vi "io_unit.vi"(0 "from_alu":T1, 1 "from_regs":T1, 2 "from_input":T1, 3 "to":T1, 4 "from":T1) -> (5 "to_alu":T2, 6 "to_regs":T2, 7 "to_output":T2)   [LabVIEW 2013]
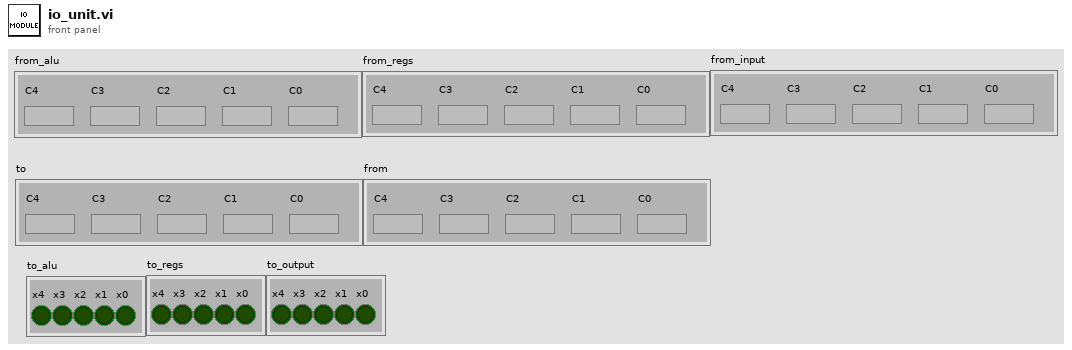
[diagram p1: front panel]
types:
  T1 = cluster{"C4":bool, "C3":bool, "C2":bool, "C1":bool, "C0":bool}
  T2 = cluster{"x4":bool, "x3":bool, "x2":bool, "x1":bool, "x0":bool}
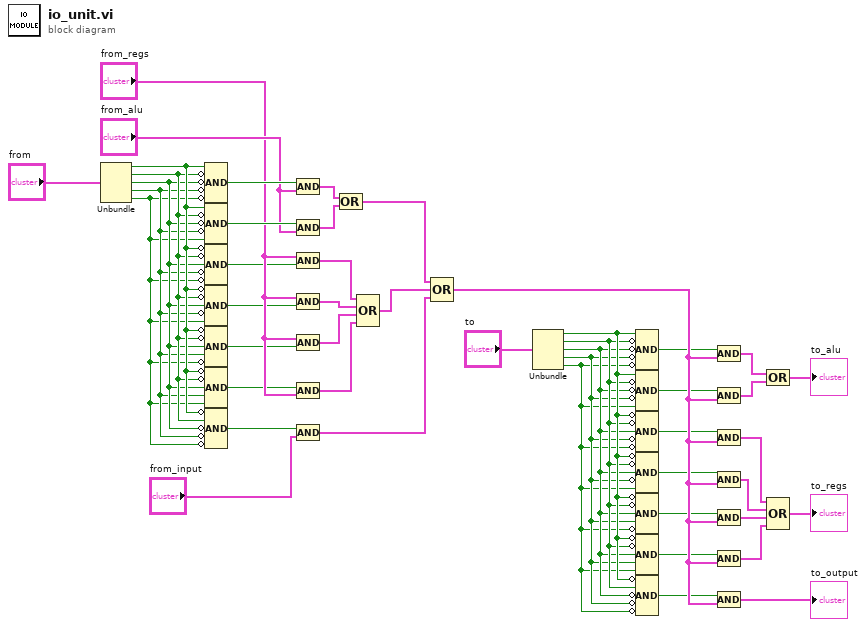
[diagram p0: block diagram]
diagram:
  n1 = Unbundle("from") -> ("C4"=w42:bool, "C3"=w41:bool, "C2"=w40:bool, "C1"=w39:bool, "C0"=w38:bool)
  n2 = Compound Arithmetic op=AND(w42, invert w41, invert w40, invert w39, invert w38) -> (w36:bool)
  n3 = Compound Arithmetic op=AND(w42, invert w41, invert w40, invert w39, w38) -> (w35:bool)
  n4 = Compound Arithmetic op=AND(invert w42, invert w41, w40, invert w39, invert w38) -> (w30:bool)
  n5 = Compound Arithmetic op=AND(invert w42, invert w41, w40, invert w39, w38) -> (w29:bool)
  n6 = Compound Arithmetic op=AND(invert w42, invert w41, w40, w39, invert w38) -> (w28:bool)
  n7 = Compound Arithmetic op=AND(invert w42, invert w41, w40, w39, w38) -> (w27:bool)
  n8 = Compound Arithmetic op=AND(invert w42, w41, invert w40, invert w39, invert w38) -> (w21:bool)
  n9 = Compound Arithmetic op=AND(w36, "from_alu") -> (w33:T1)
  n10 = Compound Arithmetic op=AND(w35, "from_alu") -> (w32:T1)
  n11 = Compound Arithmetic op=AND("from_regs", w30) -> (w26:T1)
  n12 = Compound Arithmetic op=AND("from_regs", w29) -> (w23:T1)
  n13 = Compound Arithmetic op=AND("from_regs", w28) -> (w24:T1)
  n14 = Compound Arithmetic op=AND(w27, "from_regs") -> (w25:T1)
  n15 = Compound Arithmetic op=AND(w21, "from_input") -> (w20:T1)
  n16 = Compound Arithmetic op=OR(w33, w32) -> (w18:T1)
  n17 = Compound Arithmetic op=OR(w26, w23, w24, w25) -> (w19:T1)
  n18 = Compound Arithmetic op=OR(w18, w19, w20) -> (w17:T1)
  n19 = Unbundle("to") -> ("C4"=w47:bool, "C3"=w46:bool, "C2"=w45:bool, "C1"=w44:bool, "C0"=w43:bool)
  n20 = Compound Arithmetic op=AND(w47, invert w46, invert w45, invert w44, invert w43) -> (w16:bool)
  n21 = Compound Arithmetic op=AND(w47, invert w46, invert w45, invert w44, w43) -> (w15:bool)
  n22 = Compound Arithmetic op=AND(invert w47, invert w46, w45, invert w44, invert w43) -> (w14:bool)
  n23 = Compound Arithmetic op=AND(invert w47, invert w46, w45, invert w44, w43) -> (w13:bool)
  n24 = Compound Arithmetic op=AND(invert w47, invert w46, w45, w44, invert w43) -> (w12:bool)
  n25 = Compound Arithmetic op=AND(invert w47, invert w46, w45, w44, w43) -> (w11:bool)
  n26 = Compound Arithmetic op=AND(invert w47, w46, invert w45, invert w44, invert w43) -> (w10:bool)
  n27 = Compound Arithmetic op=AND(w16, w17) -> (w3:T1)
  n28 = Compound Arithmetic op=AND(w15, w17) -> (w4:T1)
  n29 = Compound Arithmetic op=AND(w14, w17) -> (w8:T1)
  n30 = Compound Arithmetic op=AND(w13, w17) -> (w5:T1)
  n31 = Compound Arithmetic op=AND(w12, w17) -> (w6:T1)
  n32 = Compound Arithmetic op=AND(w11, w17) -> (w7:T1)
  n33 = Compound Arithmetic op=AND(w10, w17) -> (→"to_output":T1)
  n34 = Compound Arithmetic op=OR(w3, w4) -> (→"to_alu":T1)
  n35 = Compound Arithmetic op=OR(w8, w5, w6, w7) -> (→"to_regs":T1)
